vi "U3 Single Pulse Port Output (no-timer).vi"() -> ()   [LabVIEW 2021]
panel:
  in  "Starting Channel":i32=4
  in  "Pulse Type":bool=TRUE
  in  "Pulse Time (microseconds)":i32=100000
  out "Error Message":string
  out "error out":errorcluster
  # "Uses the PUT_WAIT IOType to create a single pulse on the specified digital output line\nand one higher on the U3.\n\nThe put_wait works by adding a delay between two events within a low-level Feedback\ncommand.  In the UD driver, if you add a request to set FIO0 high, add a request to wait\n100000 microseconds, add a request to set FIO0 low, and then Go, these will be sent in\na single low-level Feedback command, creating a 100 ms positive pulse on FIO0."
  # "0-7       FIO0-FIO7\n8-15     EIO0-EIO7\n16-19   CIO0-CIO3"
  # "Range is 0-8388480.\nActual resolution is 128 us.\nActual minimum is about 30 us."
  # "High Pulse\n\nLow Pulse"
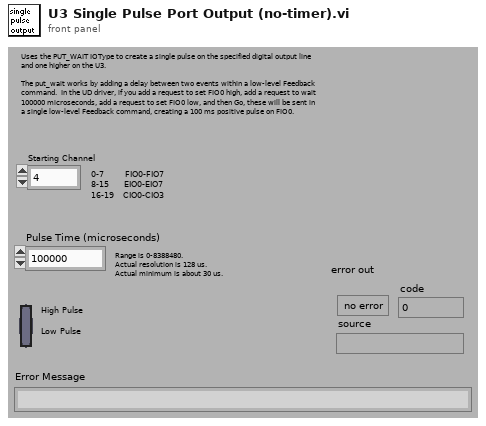
[diagram p1: front panel]
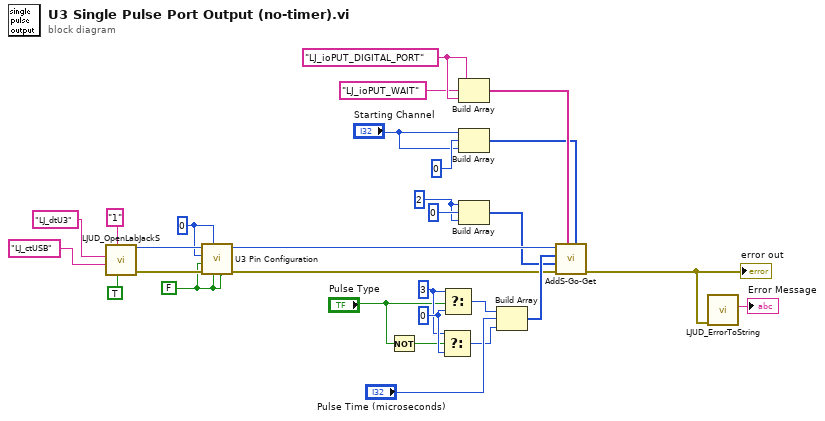
[diagram p0: block diagram]
diagram:
  w1 = 2 ("Input Element")
  w9 = 0 ("f")
  w8 = 3 ("t")
  w18 = FALSE ("Enable Counter0")
  w10 = 0 ("FIO/EIO Analog Enable")
  w17 = "LJ_ioPUT_DIGITAL_PORT" ("IOType")
  n1 = call "LJUD_OpenLabJackS.vi"("FirstFound"=TRUE, "Address"="1", "ConnectionType"="LJ_ctUSB", "DeviceType"="LJ_dtU3") -> ("error out"=w21:errorcluster, "Handle"=w22:i32)  [unwired: 5 in, 1 out]
  n2 = call "U3 Pin Configuration.vi"("Enable Counter1"=w18, "Enable Counter0"=w18, "FIO/EIO Analog Enable"=w10, "error in"=w21, "Enable DAC1"=w18, "Number of Timers Enabled"=w10, "Handle In"=w22) -> ("error out"=w20:errorcluster, "Handle Out"=w19:i32)  [unwired: 3 in]
  n3 = Not(x="Pulse Type") -> (.not. x?=w6:bool)
  n4 = Select(t=w8, s=w6, f=w9) -> (s? t:f=w4:i32)
  n5 = Select(t=w8, s="Pulse Type", f=w9) -> (s? t:f=w5:i32)
  n6 = Build Array(w17, "LJ_ioPUT_WAIT" ("Input Element"), w17) -> (w15:string[])
  n7 = Build Array("Starting Channel", 0, "Starting Channel") -> (w13:i32[])
  n8 = Build Array(w1, 0 ("Input Element"), w1) -> (w3:i32[])
  n9 = Build Array(w5, "Pulse Time (microseconds)", w4) -> (w27:i32[])
  n10 = call "AddS-Go-Get.vi"("Channels"=w13, "IOTypes"=w15, "error in"=w20, "x1"=w3, "Values Write"=w27, "Handle In"=w19) -> ("error out"=w28:errorcluster)  [unwired: 3 in, 2 out]
  "error out" <- w28
  n11 = call "LJUD_ErrorToString.vi"("error in"=w28) -> ("String"=→"Error Message":string)  [unwired: 10 in]
